vi "List Keys.vi"(8 "error in (no error)":errorcluster, 11 "SMO.Dictionary.Variant in":refnum<class "SMO.Dictionary.Variant.lvclass">) -> (0 "error out":errorcluster, 2 "Keys":string[](array[string]), 3 "SMO.Dictionary.Variant out":refnum<class "SMO.Dictionary.Variant.lvclass">)   [LabVIEW 2013, in "SMO.Dictionary.lvlib" / "SMO.Dictionary.Variant.lvclass"]
uses:
  SMO.Dictionary.Variant.lvclass
  SMO.Dictionary.Variant.lvclass/SMO.Dictionary.Variant.ctl
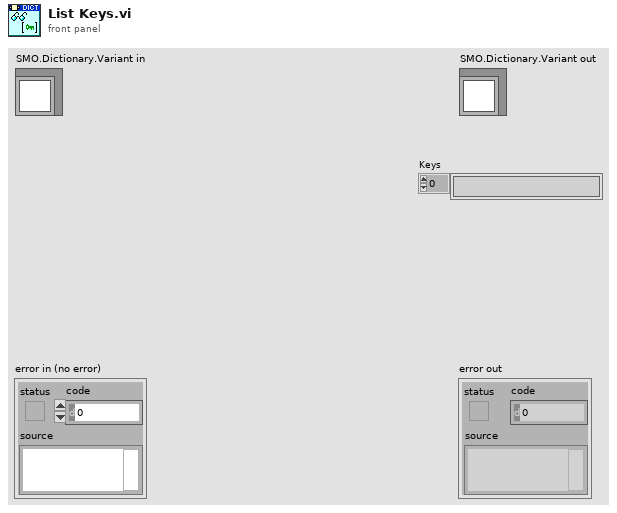
[diagram p1: front panel]
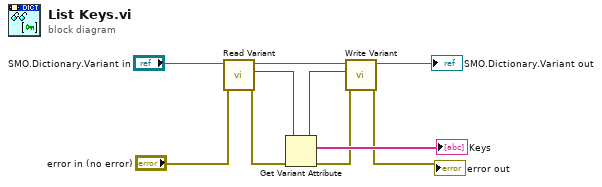
[diagram p0: block diagram]
diagram:
  n1 = call "Read Variant.vi"("error in (no error)"="error in (no error)", "SMO.Dictionary.Variant in"="SMO.Dictionary.Variant in") -> ("error out"=w3:errorcluster, "Variant"=w5:variant, "SMO.Dictionary.Variant out"=w9:refnum<class "SMO.Dictionary.Variant.lvclass">)  [unwired: 7 in]
  n2 = Get Variant Attribute(Variant=w5, error in=w3) -> (duplicate Variant=w6:variant, names=→"Keys":string[], error out=w2:errorcluster)  [unwired: 2 in, 1 out]
  n3 = call "Write Variant.vi"("error in (no error)"=w2, "Variant"=w6, "SMO.Dictionary.Variant in"=w9) -> ("error out"=→"error out":errorcluster, "SMO.Dictionary.Variant out"=→"SMO.Dictionary.Variant out":refnum<class "SMO.Dictionary.Variant.lvclass">)  [unwired: 7 in]
